vi "PicohrdlCollectSingleValueAsync.vi"(6 "Input type":i16(ring)=1 items=["Differential", "Single-Ended"], 7 "Channel in":i16=1 min=1 max=16 step=1, 8 "error in (no error)":errorcluster, 9 "Conversion time":i16(ring) items=["60ms", "100ms", "180ms", "340ms"], 10 "Voltage Range":i16(ring) items=["+/-2500mV", "+/-1200mV", "+/-625mV", "+/-312.5mV", "+/-156.25mV", "+/-78.125mV", "+/-39.0625mV"], 11 "handle in":i16) -> (0 "error out":errorcluster, 1 "channel":i16, 2 "Voltage Range out":i16(ring) items=["+/-2500mV", "+/-1200mV", "+/-625mV", "+/-312.5mV", "+/-156.25mV", "+/-78.125mV", "+/-39.0625mV"], 3 "Handle out":i16)   [LabVIEW 2010]
doc: "Calls HRDLCollectSingleValueAsync()"
uses:
  PicoHRDL.dll
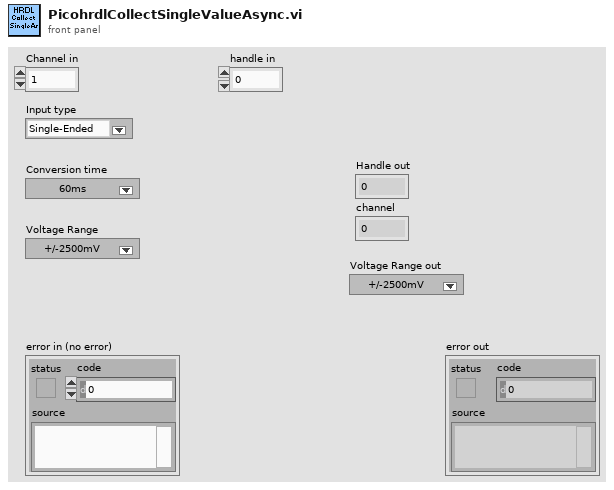
[diagram p1: front panel]
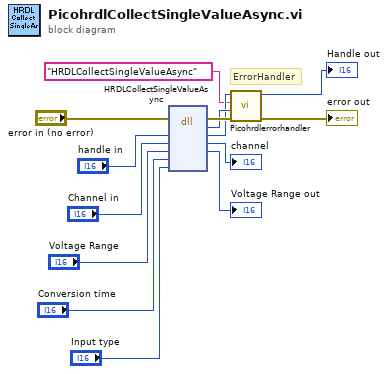
[diagram p0: block diagram]
diagram:
  # "ErrorHandler"
  n1 = dll-call lib="PicoHRDL.dll" fn="HRDLCollectSingleValueAsync"(error in="error in (no error)", "handle"="handle in", "channel"="Channel in", "range"="Voltage Range", "conversionTime"="Conversion time", "singleEnded"="Input type") -> (error out=w14:errorcluster, "return type"=w13:i16, "handle"=w12:i16, "channel"=→"channel":i16, "range"=→"Voltage Range out":i16)  [unwired: 4 in, 1 out]
  n2 = call "Picohrdlerrorhandler.vi"("Handle in"=w12, "API function"="HRDLCollectSingleValueAsync", "Return"=w13, "error in (no error)"=w14) -> ("Handle out"=→"Handle out":i16, "error out"=→"error out":errorcluster)  [unwired: 5 in]
